vi "Main.vi"(8 "error in (no error)":errorcluster, 11 "StageSPIMBase in":refnum<class "StageSPIM.lvclass">) -> (0 "error out":errorcluster, 3 "component":refnum<class "StageSPIM.lvclass">)   [LabVIEW 2012, in "StageSPIM.lvclass"]
doc: "Main VI of the component."
uses:
  StageSPIM.lvclass
  <vilib>/Distrio/Murmex/Murmex/command_enum.ctl
  StageSPIM.lvclass/StageSPIM.ctl
  <vilib>/Distrio/Murmex/InitialiseMessage/InitialiseMessage.lvclass
  <vilib>/Distrio/Murmex/GenericMessage/GenericMessage.lvclass
  <vilib>/Distrio/Murmex/TerminateMessage/TerminateMessage.lvclass
  <vilib>/Distrio/Murmex/Murmex/update_cluster.ctl
  <vilib>/Distrio/Murmex/StopMessage/StopMessage.lvclass
  <vilib>/Distrio/Murmex/ConfigureMessage/ConfigureMessage.lvclass
  <vilib>/Distrio/Murmex/Murmex/Set configure at initialise.vi
  <vilib>/Distrio/Murmex/Murmex/Set log reference.vi
  <vilib>/Distrio/Murmex/Murmex/Set VI reference.vi
  <vilib>/Distrio/Murmex/Murmex/Get ID.vi
  <vilib>/Distrio/Murmex/Murmex/Murmex.lvclass
  <vilib>/Distrio/Murmex/Message/Message.lvclass
panel:
  in  "button::stop":bool
  in  "button::configure":bool
  in  "button::quit":bool
  in  "Tab Control":enum32{"Main", "Debug"}(tab)
  in  "forwardY":bool
  in  "backY":bool
  in  "stepY":dbl[unit]
  in  "forwardZ":bool
  in  "backZ":bool
  in  "stepZ":dbl[unit]
  in  "forwardX":bool
  in  "backX":bool
  in  "stepX":dbl[unit]
  out "currentX":dbl[unit]
  out "currentY":dbl[unit]
  out "currentZ":dbl[unit]
  in  "speedZ":dbl[unit]
  in  "speedY":dbl[unit]
  in  "speedX":dbl[unit]
  in  "targetX":dbl[unit]
  in  "targetY":dbl[unit]
  in  "targetZ":dbl[unit]
  in  "button::send":bool
  out "log":string
  in  "command":T1
  in  "Generic command":string
  in  "ID":string="stage"
  out "terminate?":bool=TRUE
  # "Current\nposition"
  # "Target\nposition"
  # "Steps"
  # "Speed"
  # "X"
  # "Y"
  # "Z"
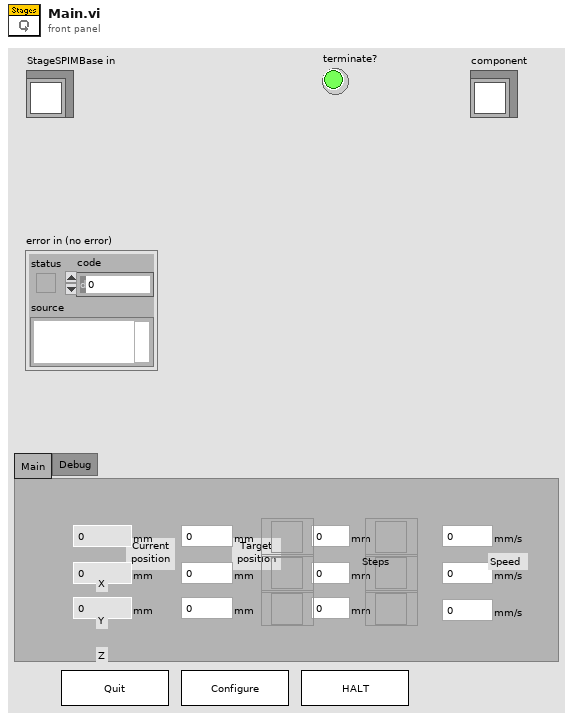
[diagram p1: front panel]
types:
  T1 = typedef "Murmex.lvlib/Murmex.lvclass/command_enum.ctl" = enum16{"null", "initialise", "reset", "terminate", "acknowledge", "update", "inspect", "inform", "proceed", "start", "stop", "fetch", "configure", "generic"}
  T2 = enum8{"Enabled", "Disabled", "Disabled and Grayed Out"}
  T3 = typedef "Murmex.lvlib/Murmex.lvclass/update_cluster.ctl" = cluster{"target ID":string, "key chains":string[], "values":variant[]}
  T4 = typedef "Murmex.lvlib/Murmex.lvclass/Event type enumerations.ctl" = enum16{"before", "after"}
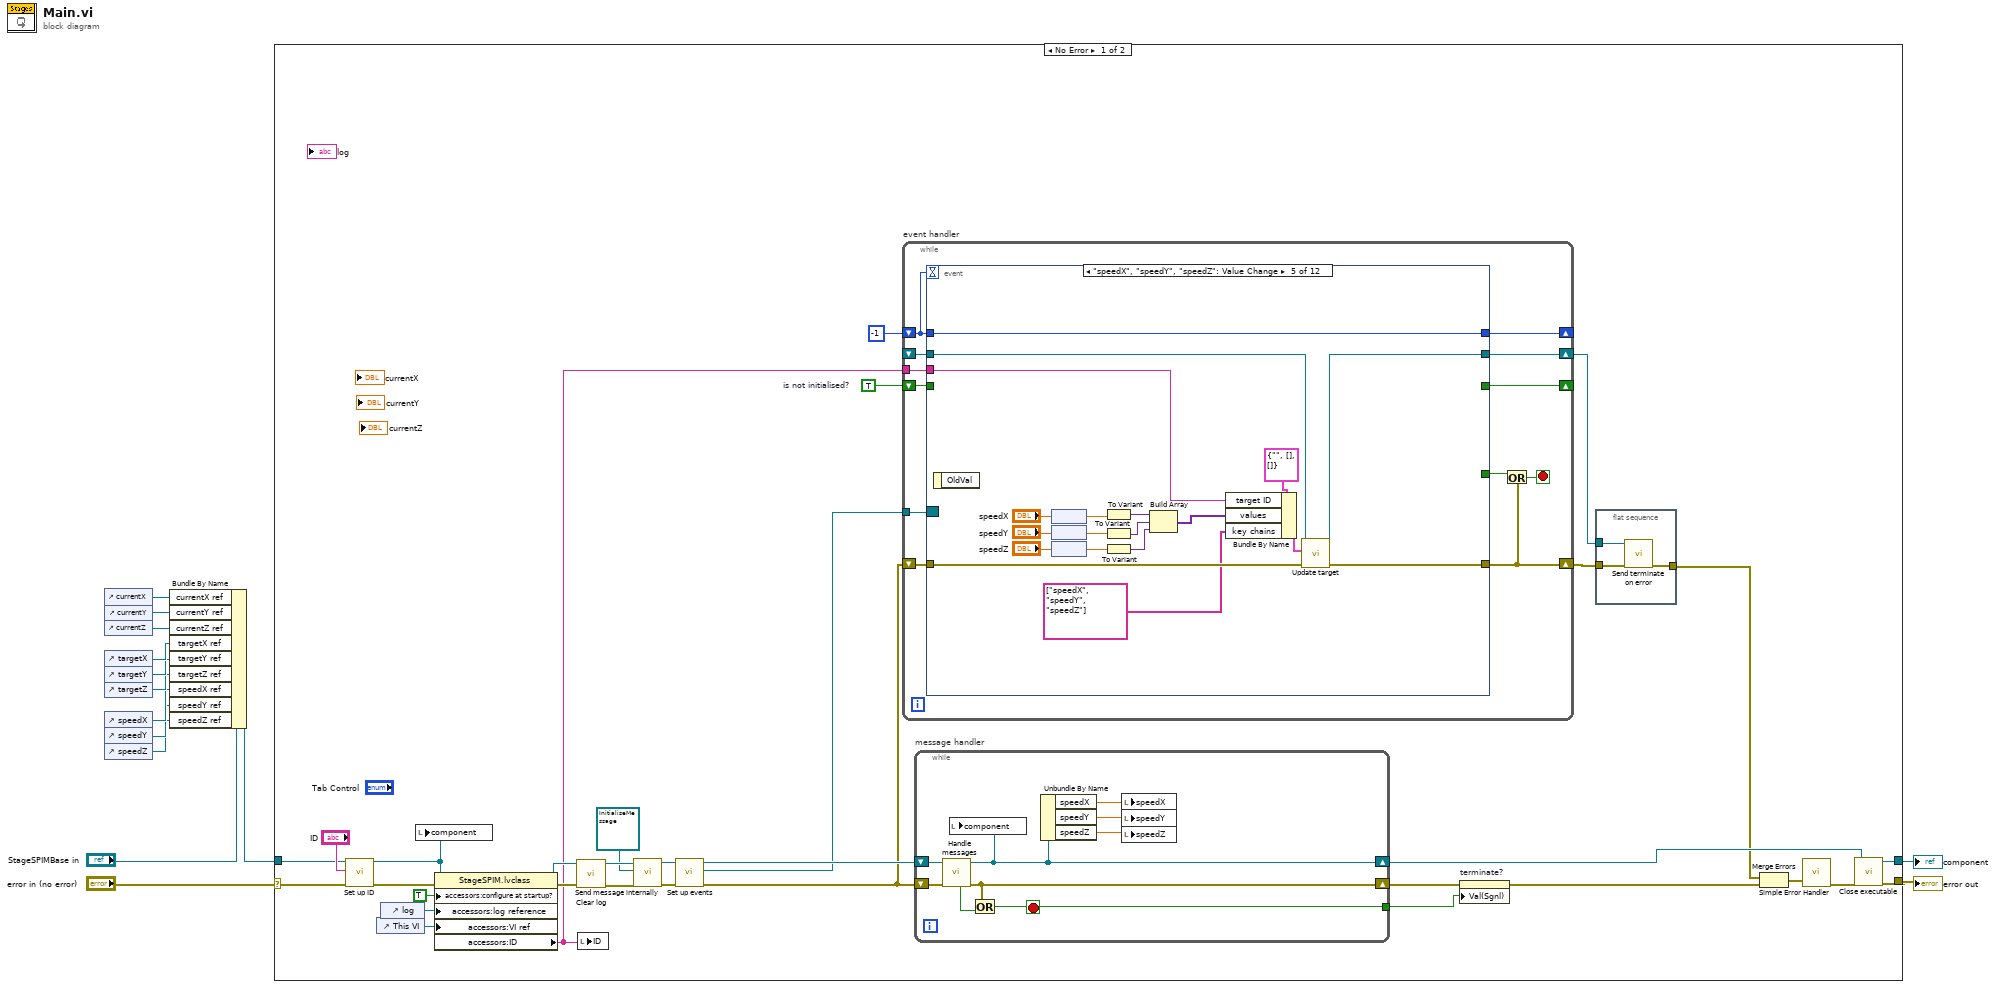
[diagram p0: block diagram]
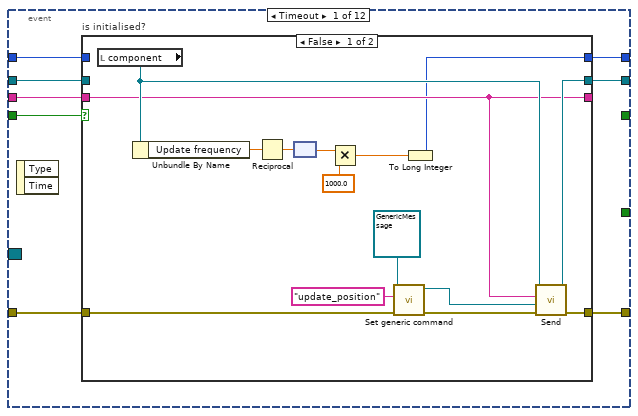
[diagram p2: hidden frame]
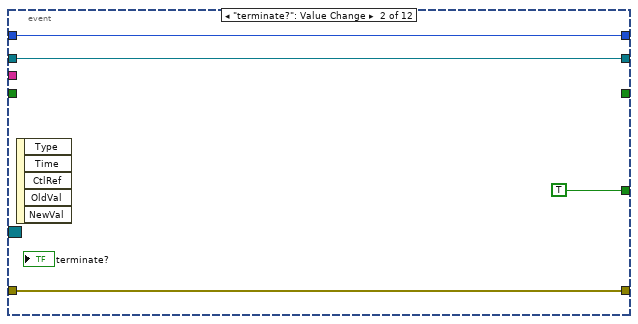
[diagram p4: hidden frame]
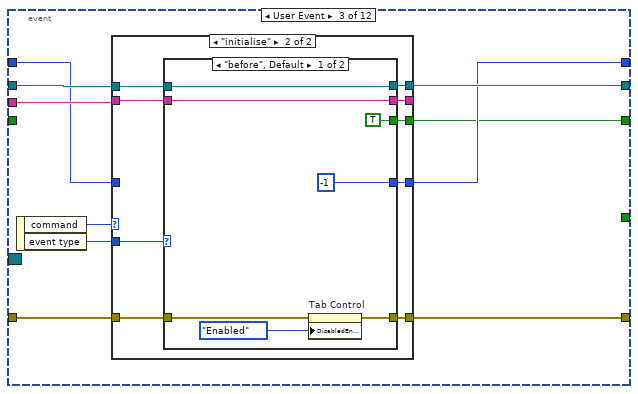
[diagram p5: hidden frame]
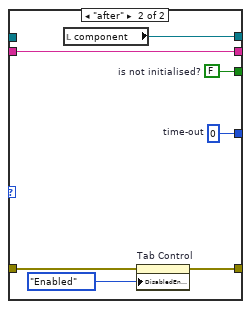
[diagram p7: hidden frame]
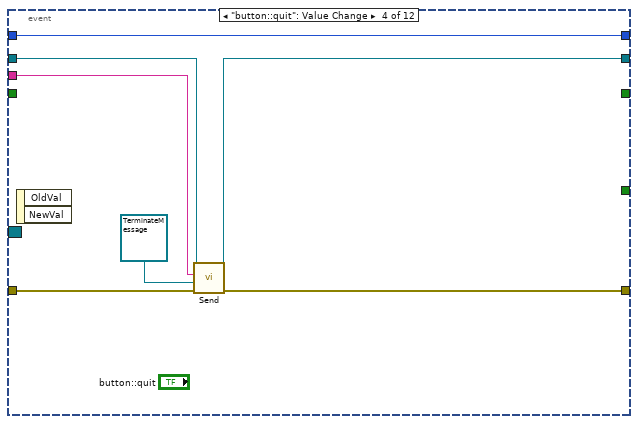
[diagram p8: hidden frame]
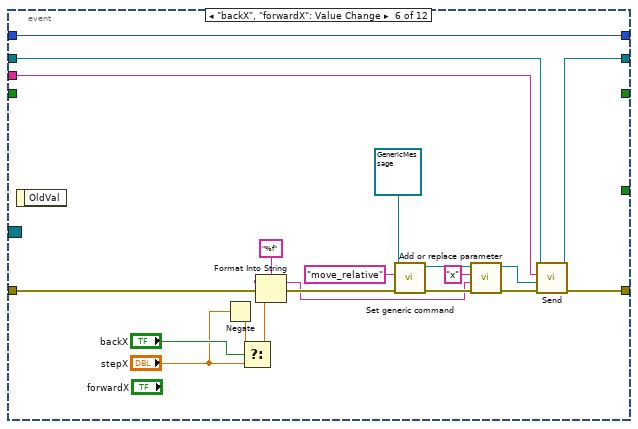
[diagram p9: hidden frame]
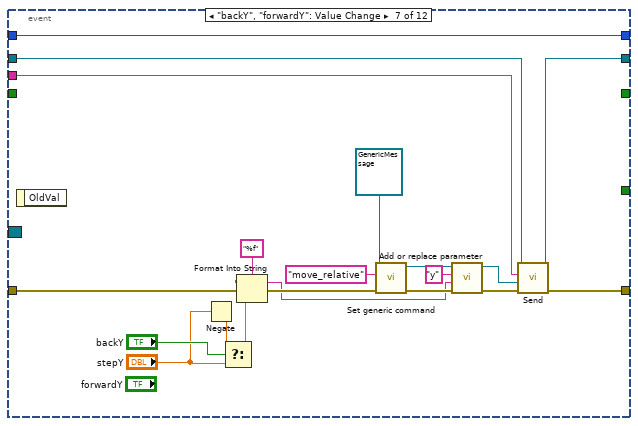
[diagram p10: hidden frame]
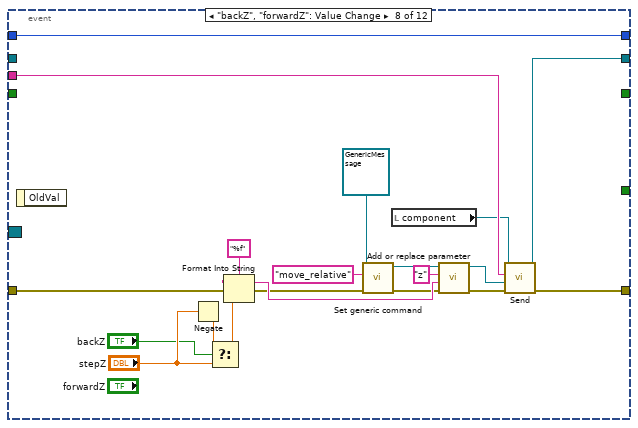
[diagram p11: hidden frame]
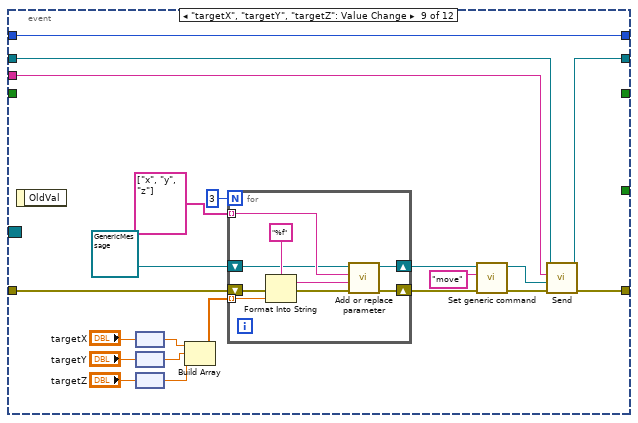
[diagram p12: hidden frame]
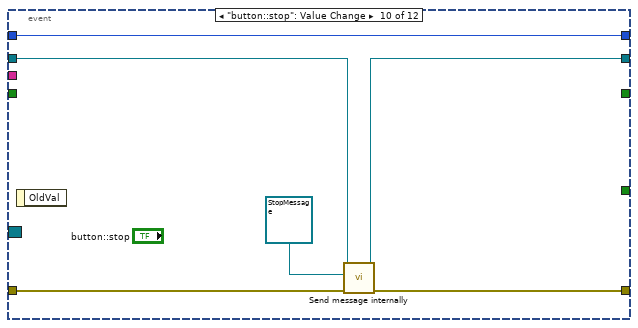
[diagram p13: hidden frame]
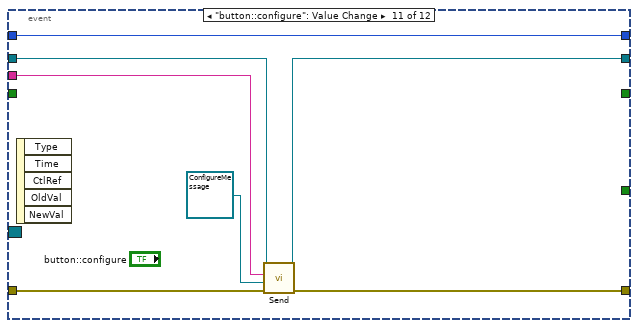
[diagram p14: hidden frame]
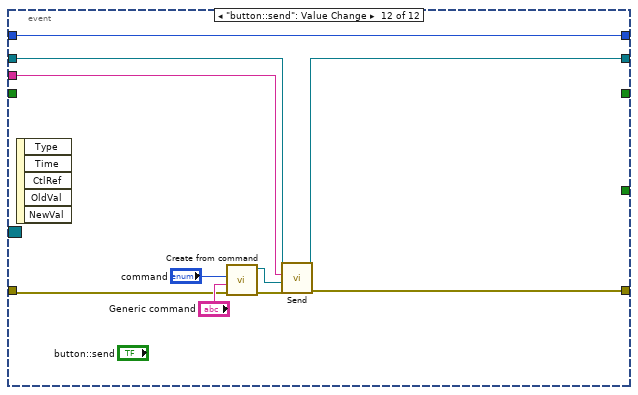
[diagram p15: hidden frame]
diagram:
  n1 = control-ref of="currentX"() -> (w9:refnum<vi>)
  n2 = control-ref of="currentY"() -> (w8:refnum<vi>)
  n3 = control-ref of="currentZ"() -> (w7:refnum<vi>)
  n4 = control-ref of="targetX"() -> (w6:refnum<vi>)
  n5 = control-ref of="targetY"() -> (w5:refnum<vi>)
  n6 = control-ref of="targetZ"() -> (w4:refnum<vi>)
  n7 = control-ref of="speedX"() -> (w3:refnum<vi>)
  n8 = control-ref of="speedY"() -> (w2:refnum<vi>)
  n9 = control-ref of="speedZ"() -> (w1:refnum<vi>)
  n10 = Bundle By Name(cluster="StageSPIMBase in", "currentX ref"=w9, "currentY ref"=w8, "currentZ ref"=w7, "targetX ref"=w6, "targetY ref"=w5, "targetZ ref"=w4, "speedX ref"=w3, "speedY ref"=w2, "speedZ ref"=w1) -> (w12:refnum<class "StageSPIM.lvclass">)
  n11 = case shown="No Error" "error in (no error)" {
    selector: "error in (no error)" -> [w45 w278]
    tunnel: w12 -> [w44 w279]
    tunnel: [w29 w278] -> w11
    tunnel: [w27 w279] -> w10
    frame No Error {
      w19 = TRUE  # is not initialised?
      n12 = call <vilib>:"Set up ID.vi"("error in (no error)"=w45, "component ID"="ID", "MurmexBase in"=w44) -> ("error out"=w43:errorcluster, "MurmexBase out"=w20:refnum<class "StageSPIM.lvclass">)  [unwired: 6 in, 1 out]
      n13 = control-ref of="This VI"() -> (w40:refnum<vi>)
      n14 = control-ref of="log"() -> (w41:refnum<vi>)
      n15 = local write "component"(w20) -> ()
      n16 = property class="StageSPIM.lvclass"(reference=w20, error in=w43, "accessors:configure at startup?"=TRUE ("configure at startup?"), "accessors:log reference"=w41, "accessors:VI ref"=w40) -> (reference out=w38:refnum<class "StageSPIM.lvclass">, error out=w39:errorcluster, "accessors:ID"=w21:string)
      n17 = call <vilib>:"Clear log.vi"("error in (no error)"=w39, "MurmexBase in"=w38) -> ("error out"=w37:errorcluster, "MurmexBase out"=w36:refnum<class "StageSPIM.lvclass">)  [unwired: 8 in]
      n18 = local write "ID"(w21) -> ()
      n19 = call <vilib>:"Send message internally.vi"("error in (no error)"=w37, "Message"=refnum<class "InitialiseMessage.lvclass"> refnum ("Distrio Murmex 1.1:InitialiseMessage"), "Murmex in"=w36) -> ("error out"=w34:errorcluster, "Murmex out"=w33:refnum<class "StageSPIM.lvclass">)  [unwired: 7 in]
      n20 = call <vilib>:"Set up events.vi"("error in (no error)"=w34, "MurmexBase in"=w33) -> ("error out"=w26:errorcluster, "Event Registration Refnum"=w25:refnum<event-registration>, "MurmexBase out"=w32:refnum<class "StageSPIM.lvclass">)  [unwired: 7 in]
      n21 = while "event handler" {
        shift-right: [w52] -> w23
        shift-left: w26 -> [w61]
        tunnel: w25 -> [w60]
        shift-right: [w58] -> _
        shift-left: -1 -> [w59]
        shift-right: [w55] -> w15
        shift-left: _ -> [w54]
        shift-right: [w50] -> _
        shift-left: w19 -> [w51]
        tunnel: w21 -> [w56]
        stop <- w57 stop-if-true
        n22 = event shown="[4] \"speedX\", \"speedY\", \"speedZ\": Value Change" {
          selector: w60 -> [_ _ _ _ _ _ _ _ _ _ _ _]
          dyn-events: _ -> [_ _ _ _ _ _ _ _ _ _ _ _]
          timeout: w59 -> [_ _ _ _ _ _ _ _ _ _ _ _]
          tunnel: w61 -> [w68 w92 w102 w135 w153 w157 w179 w199 w216 w251 w258 w264]
          tunnel: w59 -> [w62 w90 w94 w130 w140 w156 w178 w200 w231 w249 w252 w260]
          tunnel: [w69 w90 w95 w130 w140 w156 w178 w200 w231 w249 w252 w260] -> w58
          tunnel: [w67 w92 w96 w134 w152 w163 w183 w202 w235 w247 w257 w263] -> w52
          tunnel: w56 -> [w66 _ w99 w131 w151 w160 w180 w201 w232 _ w255 w259]
          tunnel: w54 -> [w64 w89 w98 w133 w150 w161 w181 _ w233 w250 w254 w262]
          tunnel: [w65 w89 w97 w132 w149 w162 w182 w203 w234 w248 w253 w261] -> w55
          tunnel: [_ TRUE _ _ _ _ _ _ _ _ _ _] -> w53
          tunnel: w51 -> [w63 _ _ _ _ _ _ _ _ _ _ _]
          tunnel: [_ _ w93 _ _ _ _ _ _ _ _ _] -> w50
          event Timeout {
            n23 = event-data() -> ()  [unwired: 1 in, 2 out]
            n24 = case "is initialised?" shown="False" w63 {
              tunnel: [w70 w85] -> w69
              tunnel: w68 -> [w78 w88]
              tunnel: [w77 w88] -> w67
              tunnel: w66 -> [w73 w87]
              tunnel: [w75 w86] -> w65
              tunnel: w64 -> [_ w86]
              tunnel: [w73 w87] -> _
              tunnel: w62 -> [_ w85]
              frame False {
                n25 = local read "component"() -> (w74:refnum<class "StageSPIM.lvclass">)
                n26 = Unbundle By Name(w74) -> ("Update frequency"=w84:dbl[unit])
                n27 = Reciprocal(x=w84) -> (1/x=w83:dbl[unit])
                n28 = node(w83) -> (w72:dbl)
                n29 = Multiply(x=w72, y=1000.0) -> (x*y=w71:dbl)
                n30 = call <vilib>:"Set generic command.vi"("error in (no error)"=w78, "generic command"="update_position", "GenericMessage in"=refnum<class "GenericMessage.lvclass"> refnum ("Distrio Murmex 1.1:GenericMessage")) -> ("error out"=w79:errorcluster, "GenericMessage out"=w76:refnum<class "GenericMessage.lvclass">)  [unwired: 7 in]
                n31 = To Long Integer(number=w71) -> (32bit integer=w70:i32)
                n32 = call <vilib>:"Send.vi"("error in (no error)"=w79, "Message"=w76, "recipient"=w73, "Murmex in"=w74) -> ("error out"=w77:errorcluster, "Murmex out"=w75:refnum<class "StageSPIM.lvclass">)  [unwired: 6 in]
              }
              frame True {
              }
            }
          }
          event "terminate?": Value Change {
            n33 = event-data() -> ()  [unwired: 1 in, 5 out]
          }
          event User Event {
            n34 = event-data() -> ("command"=w101:T1, "event type"=w100:T4)  [unwired: 1 in]
            n35 = case shown="\"initialise\"" w101 {
              tunnel: w102 -> [w104 w115]
              tunnel: [w104 w114] -> w96
              tunnel: w99 -> [w106 w113]
              tunnel: [w105 w112] -> w97
              tunnel: w98 -> [w105 w111]
              tunnel: [w106 w110] -> _
              tunnel: w100 -> [_ w109]
              tunnel: [w103 w108] -> w95
              tunnel: w94 -> [w103 _]
              tunnel: [_ w107] -> w93
              frame "null", Default {
              }
              frame "initialise" {
                n36 = case shown="\"before\", Default" w109 {
                  tunnel: [w121 w128] -> w114
                  tunnel: w115 -> [w122 w129]
                  tunnel: w113 -> [w119 w125]
                  tunnel: [w118 w127] -> w112
                  tunnel: w111 -> [w118 _]
                  tunnel: [w119 w125] -> w110
                  tunnel: [-1 w124] -> w108
                  tunnel: [TRUE ("is not initialised?") w123] -> w107
                  frame "before", Default {
                    n37 = property on="Tab Control" class="TabCtl (strict)"(error in=w122, "DisabledEnum"=T2."Enabled" ("Disabled")) -> (error out=w121:errorcluster)  [unwired: 1 in, 1 out]
                  }
                  frame "after" {
                    w123 = FALSE  # is not initialised?
                    w124 = 0  # time-out
                    n38 = local read "component"() -> (w127:refnum<class "StageSPIM.lvclass">)
                    n39 = property on="Tab Control" class="TabCtl (strict)"(error in=w129, "DisabledEnum"=T2."Enabled" ("Disabled")) -> (error out=w128:errorcluster)  [unwired: 1 in, 1 out]
                  }
                }
              }
            }
          }
          event "button::quit": Value Change {
            n40 = event-data() -> ()  [unwired: 1 in, 2 out]
            n41 = call <vilib>:"Send.vi"("error in (no error)"=w135, "Message"=refnum<class "TerminateMessage.lvclass"> refnum ("Murmex.lvlib:TerminateMessage"), "recipient"=w131, "Murmex in"=w133) -> ("error out"=w134:errorcluster, "Murmex out"=w132:refnum<class "StageSPIM.lvclass">)  [unwired: 6 in]
          }
          event "speedX", "speedY", "speedZ": Value Change {
            n42 = event-data() -> ()  [unwired: 1 in, 1 out]
            n43 = node("speedX") -> (w137:dbl)
            n44 = node("speedY") -> (w138:dbl)
            n45 = node("speedZ") -> (w139:dbl)
            n46 = To Variant(anything=w137) -> (Variant=w145:variant)
            n47 = To Variant(anything=w138) -> (Variant=w144:variant)
            n48 = To Variant(anything=w139) -> (Variant=w143:variant)
            n49 = Build Array(w145, w144, w143) -> (w142:variant[])
            n50 = Bundle By Name(cluster=T3 {"target ID"="", "key chains"=[], "values"=[]} ("update cluster"), "target ID"=w151, "values"=w142, "key chains"=string[] ["speedX", "speedY", "speedZ"]) -> (w155:T3)
            n51 = call <vilib>:"Update target.vi"("error in (no error)"=w153, "update cluster"=w155, "MurmexBase in"=w150) -> ("error out"=w152:errorcluster, "MurmexBase out"=w149:refnum<class "StageSPIM.lvclass">)  [unwired: 7 in]
          }
          event "backX", "forwardX": Value Change {
            n52 = event-data() -> ()  [unwired: 1 in, 1 out]
            n53 = Negate(x="stepX") -> (-x=w170:dbl[unit])
            n54 = Select(t=w170, s="backX", f="stepX") -> (s? t:f=w165:dbl[unit])
            n55 = Format Into String(format string="%f", error in=w157, w165) -> (resulting string=w166:string, error out=w169:errorcluster)  [unwired: 1 in]
            n56 = call <vilib>:"Set generic command.vi"("error in (no error)"=w169, "generic command"="move_relative", "GenericMessage in"=refnum<class "GenericMessage.lvclass"> refnum ("Distrio Murmex 1.1:GenericMessage")) -> ("error out"=w174:errorcluster, "GenericMessage out"=w172:refnum<class "GenericMessage.lvclass">)  [unwired: 7 in]
            n57 = call <vilib>:"Add or replace parameter.vi"("error in (no error)"=w174, "value"=w166, "name"="x", "Message in"=w172) -> ("error out"=w173:errorcluster, "Message out"=w167:refnum<class "GenericMessage.lvclass">)  [unwired: 6 in]
            n58 = call <vilib>:"Send.vi"("error in (no error)"=w173, "Message"=w167, "recipient"=w160, "Murmex in"=w161) -> ("error out"=w163:errorcluster, "Murmex out"=w162:refnum<class "StageSPIM.lvclass">)  [unwired: 6 in]
          }
          event "backY", "forwardY": Value Change {
            n59 = event-data() -> ()  [unwired: 1 in, 1 out]
            n60 = Negate(x="stepY") -> (-x=w190:dbl[unit])
            n61 = Select(t=w190, s="backY", f="stepY") -> (s? t:f=w185:dbl[unit])
            n62 = Format Into String(format string="%f", error in=w179, w185) -> (resulting string=w186:string, error out=w189:errorcluster)  [unwired: 1 in]
            n63 = call <vilib>:"Set generic command.vi"("error in (no error)"=w189, "generic command"="move_relative", "GenericMessage in"=refnum<class "GenericMessage.lvclass"> refnum ("Distrio Murmex 1.1:GenericMessage")) -> ("error out"=w194:errorcluster, "GenericMessage out"=w192:refnum<class "GenericMessage.lvclass">)  [unwired: 7 in]
            n64 = call <vilib>:"Add or replace parameter.vi"("error in (no error)"=w194, "value"=w186, "name"="y", "Message in"=w192) -> ("error out"=w193:errorcluster, "Message out"=w187:refnum<class "GenericMessage.lvclass">)  [unwired: 6 in]
            n65 = call <vilib>:"Send.vi"("error in (no error)"=w193, "Message"=w187, "recipient"=w180, "Murmex in"=w181) -> ("error out"=w183:errorcluster, "Murmex out"=w182:refnum<class "StageSPIM.lvclass">)  [unwired: 6 in]
          }
          event "backZ", "forwardZ": Value Change {
            n66 = event-data() -> ()  [unwired: 1 in, 1 out]
            n67 = Negate(x="stepZ") -> (-x=w209:dbl[unit])
            n68 = Select(t=w209, s="backZ", f="stepZ") -> (s? t:f=w214:dbl[unit])
            n69 = Format Into String(format string="%f", error in=w199, w214) -> (resulting string=w213:string, error out=w210:errorcluster)  [unwired: 1 in]
            n70 = call <vilib>:"Set generic command.vi"("error in (no error)"=w210, "generic command"="move_relative", "GenericMessage in"=refnum<class "GenericMessage.lvclass"> refnum ("Distrio Murmex 1.1:GenericMessage")) -> ("error out"=w205:errorcluster, "GenericMessage out"=w207:refnum<class "GenericMessage.lvclass">)  [unwired: 7 in]
            n71 = local read "component"() -> (w196:refnum<class "StageSPIM.lvclass">)
            n72 = call <vilib>:"Add or replace parameter.vi"("error in (no error)"=w205, "value"=w213, "name"="z", "Message in"=w207) -> ("error out"=w206:errorcluster, "Message out"=w212:refnum<class "GenericMessage.lvclass">)  [unwired: 6 in]
            n73 = call <vilib>:"Send.vi"("error in (no error)"=w206, "Message"=w212, "recipient"=w201, "Murmex in"=w196) -> ("error out"=w202:errorcluster, "Murmex out"=w203:refnum<class "StageSPIM.lvclass">)  [unwired: 6 in]
          }
          event "targetX", "targetY", "targetZ": Value Change {
            n74 = event-data() -> ()  [unwired: 1 in, 1 out]
            n75 = node("targetX") -> (w222:dbl)
            n76 = node("targetY") -> (w218:dbl)
            n77 = node("targetZ") -> (w219:dbl)
            n78 = Build Array(w222, w218, w219) -> (w217:dbl[])
            n79 = for {
              N: 3 -> [_]
              shift-right: [w243] -> w228
              shift-left: w216 -> [w242]
              tunnel: string[] ["x", "y", "z"] -> [w241] mode=indexing
              shift-right: [w239] -> w224
              shift-left: refnum<class "GenericMessage.lvclass"> refnum ("Distrio Murmex 1.1:GenericMessage") -> [w240]
              tunnel: w217 -> [w238] mode=indexing
              n80 = Format Into String(format string="%f", error in=w242, w238) -> (resulting string=w237:string, error out=w244:errorcluster)  [unwired: 1 in]
              n81 = call <vilib>:"Add or replace parameter.vi"("error in (no error)"=w244, "value"=w237, "name"=w241, "Message in"=w240) -> ("error out"=w243:errorcluster, "Message out"=w239:refnum<class "GenericMessage.lvclass">)  [unwired: 6 in]
            }
            n82 = call <vilib>:"Set generic command.vi"("error in (no error)"=w228, "generic command"="move", "GenericMessage in"=w224) -> ("error out"=w230:errorcluster, "GenericMessage out"=w229:refnum<class "GenericMessage.lvclass">)  [unwired: 7 in]
            n83 = call <vilib>:"Send.vi"("error in (no error)"=w230, "Message"=w229, "recipient"=w232, "Murmex in"=w233) -> ("error out"=w235:errorcluster, "Murmex out"=w234:refnum<class "StageSPIM.lvclass">)  [unwired: 6 in]
          }
          event "button::stop": Value Change {
            n84 = event-data() -> ()  [unwired: 1 in, 1 out]
            n85 = call <vilib>:"Send message internally.vi"("error in (no error)"=w251, "Message"=refnum<class "StopMessage.lvclass"> refnum ("Distrio Murmex 1.5:StopMessage"), "Murmex in"=w250) -> ("error out"=w247:errorcluster, "Murmex out"=w248:refnum<class "StageSPIM.lvclass">)  [unwired: 7 in]
          }
          event "button::configure": Value Change {
            n86 = event-data() -> ()  [unwired: 1 in, 5 out]
            n87 = call <vilib>:"Send.vi"("error in (no error)"=w258, "Message"=refnum<class "ConfigureMessage.lvclass"> refnum ("Distrio Murmex 1.1:ConfigureMessage"), "recipient"=w255, "Murmex in"=w254) -> ("error out"=w257:errorcluster, "Murmex out"=w253:refnum<class "StageSPIM.lvclass">)  [unwired: 6 in]
          }
          event "button::send": Value Change {
            n88 = event-data() -> ()  [unwired: 1 in, 5 out]
            n89 = call <vilib>:"Create from command.vi"("error in (no error)"=w264, "generic command"="Generic command", "command"="command") -> ("error out"=w266:errorcluster, "Message out"=w267:refnum<class "Message.lvclass">)  [unwired: 7 in]
            n90 = call <vilib>:"Send.vi"("error in (no error)"=w266, "Message"=w267, "recipient"=w259, "Murmex in"=w262) -> ("error out"=w263:errorcluster, "Murmex out"=w261:refnum<class "StageSPIM.lvclass">)  [unwired: 6 in]
          }
        }
        n91 = Or(x=w53, y=w52) -> (x .or. y?=w57:bool)
      }
      n92 = while "message handler" {
        shift-right: [w275] -> w18
        shift-left: w26 -> [w277]
        shift-right: [w272] -> w28
        shift-left: w32 -> [w276]
        tunnel: [w273] -> w16
        stop <- w273 stop-if-true
        n93 = call <vilib>:"Handle messages.vi"("error in (no error)"=w277, "Murmex in"=w276) -> ("error out"=w275:errorcluster, "Murmex out"=w272:refnum<class "StageSPIM.lvclass">, "terminated?"=w274:bool)  [unwired: 7 in]
        n94 = local write "component"(w272) -> ()
        n95 = Or(x=w275, y=w274) -> (x .or. y?=w273:bool)
        n96 = Unbundle By Name(w272) -> ("speedX"=w271:dbl[unit], "speedY"=w270:dbl[unit], "speedZ"=w269:dbl[unit])
        n97 = local write "speedX"(w271) -> ()
        n98 = local write "speedY"(w270) -> ()
        n99 = local write "speedZ"(w269) -> ()
      }
      n100 = property on="terminate?" class="Bool (strict)"(error in=w18, "Val(Sgnl)"=w16) -> (error out=w17:errorcluster)  [unwired: 1 in, 1 out]
      n101 = flat-sequence {
        tunnel: w23 -> [w49]
        tunnel: [w48] -> w22
        tunnel: w15 -> [w47]
        frame #0 {
          n102 = call <vilib>:"Send terminate on error.vi"("error in (no error)"=w49, "Murmex in"=w47) -> ("error out"=w48:errorcluster)  [unwired: 8 in, 1 out]
        }
      }
      n103 = Merge Errors(w22, w17) -> (w31:errorcluster)
      n104 = call <vilib>:"Simple Error Handler.vi"("error in (no error)"=w31) -> ("error out"=w30:errorcluster)  [unwired: 4 in, 4 out]
      n105 = call <vilib>:"Close executable.vi"("error in (no error)"=w30, "MurmexBase in"=w28) -> ("error out"=w29:errorcluster, "MurmexBase out"=w27:refnum<class "StageSPIM.lvclass">)  [unwired: 8 in]
    }
    frame Error {
    }
  }
  "error out" <- w11
  "component" <- w10
